vi "FL_Make_RAW_data_frame_and_put_to_queue.vi"(8 "error in":errorcluster, 10 "Queue in":refnum<queue>, 11 "VISA resource name in":refnum<visa-resource-name>) -> (0 "error out":errorcluster, 2 "Queue out":refnum<queue>, 3 "VISA resource name out":refnum<visa-resource-name>)   [LabVIEW 2018]
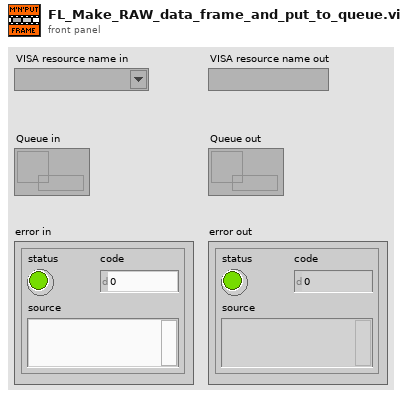
[diagram p1: front panel]
types:
  T1 = cluster{"read buffer":string, "seconds since 1Jan1904":timestamp}
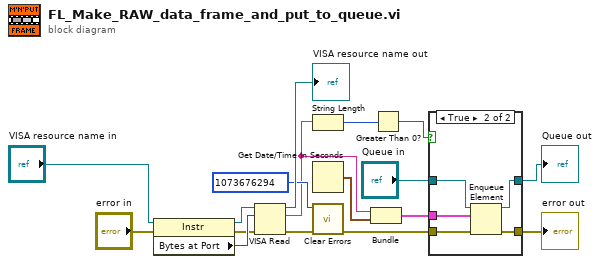
[diagram p0: block diagram]
diagram:
  n1 = property class="Instr"(reference="VISA resource name in", error in="error in") -> (reference out=w3:refnum<visa-resource-name>, error out=w4:errorcluster, "Bytes at Port"=w5:u32)
  n2 = VISA Read(VISA resource name=w3, byte count=w5, error in (no error)=w4) -> (VISA resource name out=→"VISA resource name out":refnum<visa-resource-name>, read buffer=w1:string, error out=w7:errorcluster)  [unwired: 1 out]
  n3 = String Length(string=w1) -> (length=w12:i32)
  n4 = Get Date/Time In Seconds ("Current time")() -> (seconds since 1Jan1904=w11:timestamp)
  n5 = call <vilib>:"Clear Errors.vi"("error in (no error)"=w7, "specific error code to clear (0: all)"=1073676294) -> ("error out"=w16:errorcluster)  [unwired: 4 in, 1 out]
  n6 = Bundle("read buffer"=w1, "seconds since 1Jan1904"=w11) -> (w15:T1)  [unwired: 1 in]
  n7 = Greater Than 0?(x=w12) -> (x > 0?=w17:bool)
  n8 = case shown="True" w17 {
    tunnel: w15 -> [_ w20]
    tunnel: w16 -> [w19 w22]
    tunnel: [w19 w21] -> w8
    tunnel: "Queue in" -> [w18 w24]
    tunnel: [w18 w23] -> w10
    frame False {
    }
    frame True {
      n9 = Enqueue Element(queue=w24, element=w20, error in (no error)=w22) -> (queue out=w23:refnum<queue>, error out=w21:errorcluster)  [unwired: 1 in, 1 out]
    }
  }
  "Queue out" <- w10
  "error out" <- w8
